vi "PlotBandsAgainstRun.vi"(8 "Bands?":bool, 11 "Graph":refnum<vi>) -> ()   [LabVIEW 2022 SP3]
panel:
  in  "Matlab":bool
  in  "Files":i32(listbox)
  in  "Stop Button":bool
  out "Data 2":cluster{dbl, "dt":dbl, "Y":dbl[]}[](graph)
  out "lines":i32
  out "Data":cluster{dbl, dbl, dbl[]}[](graph)
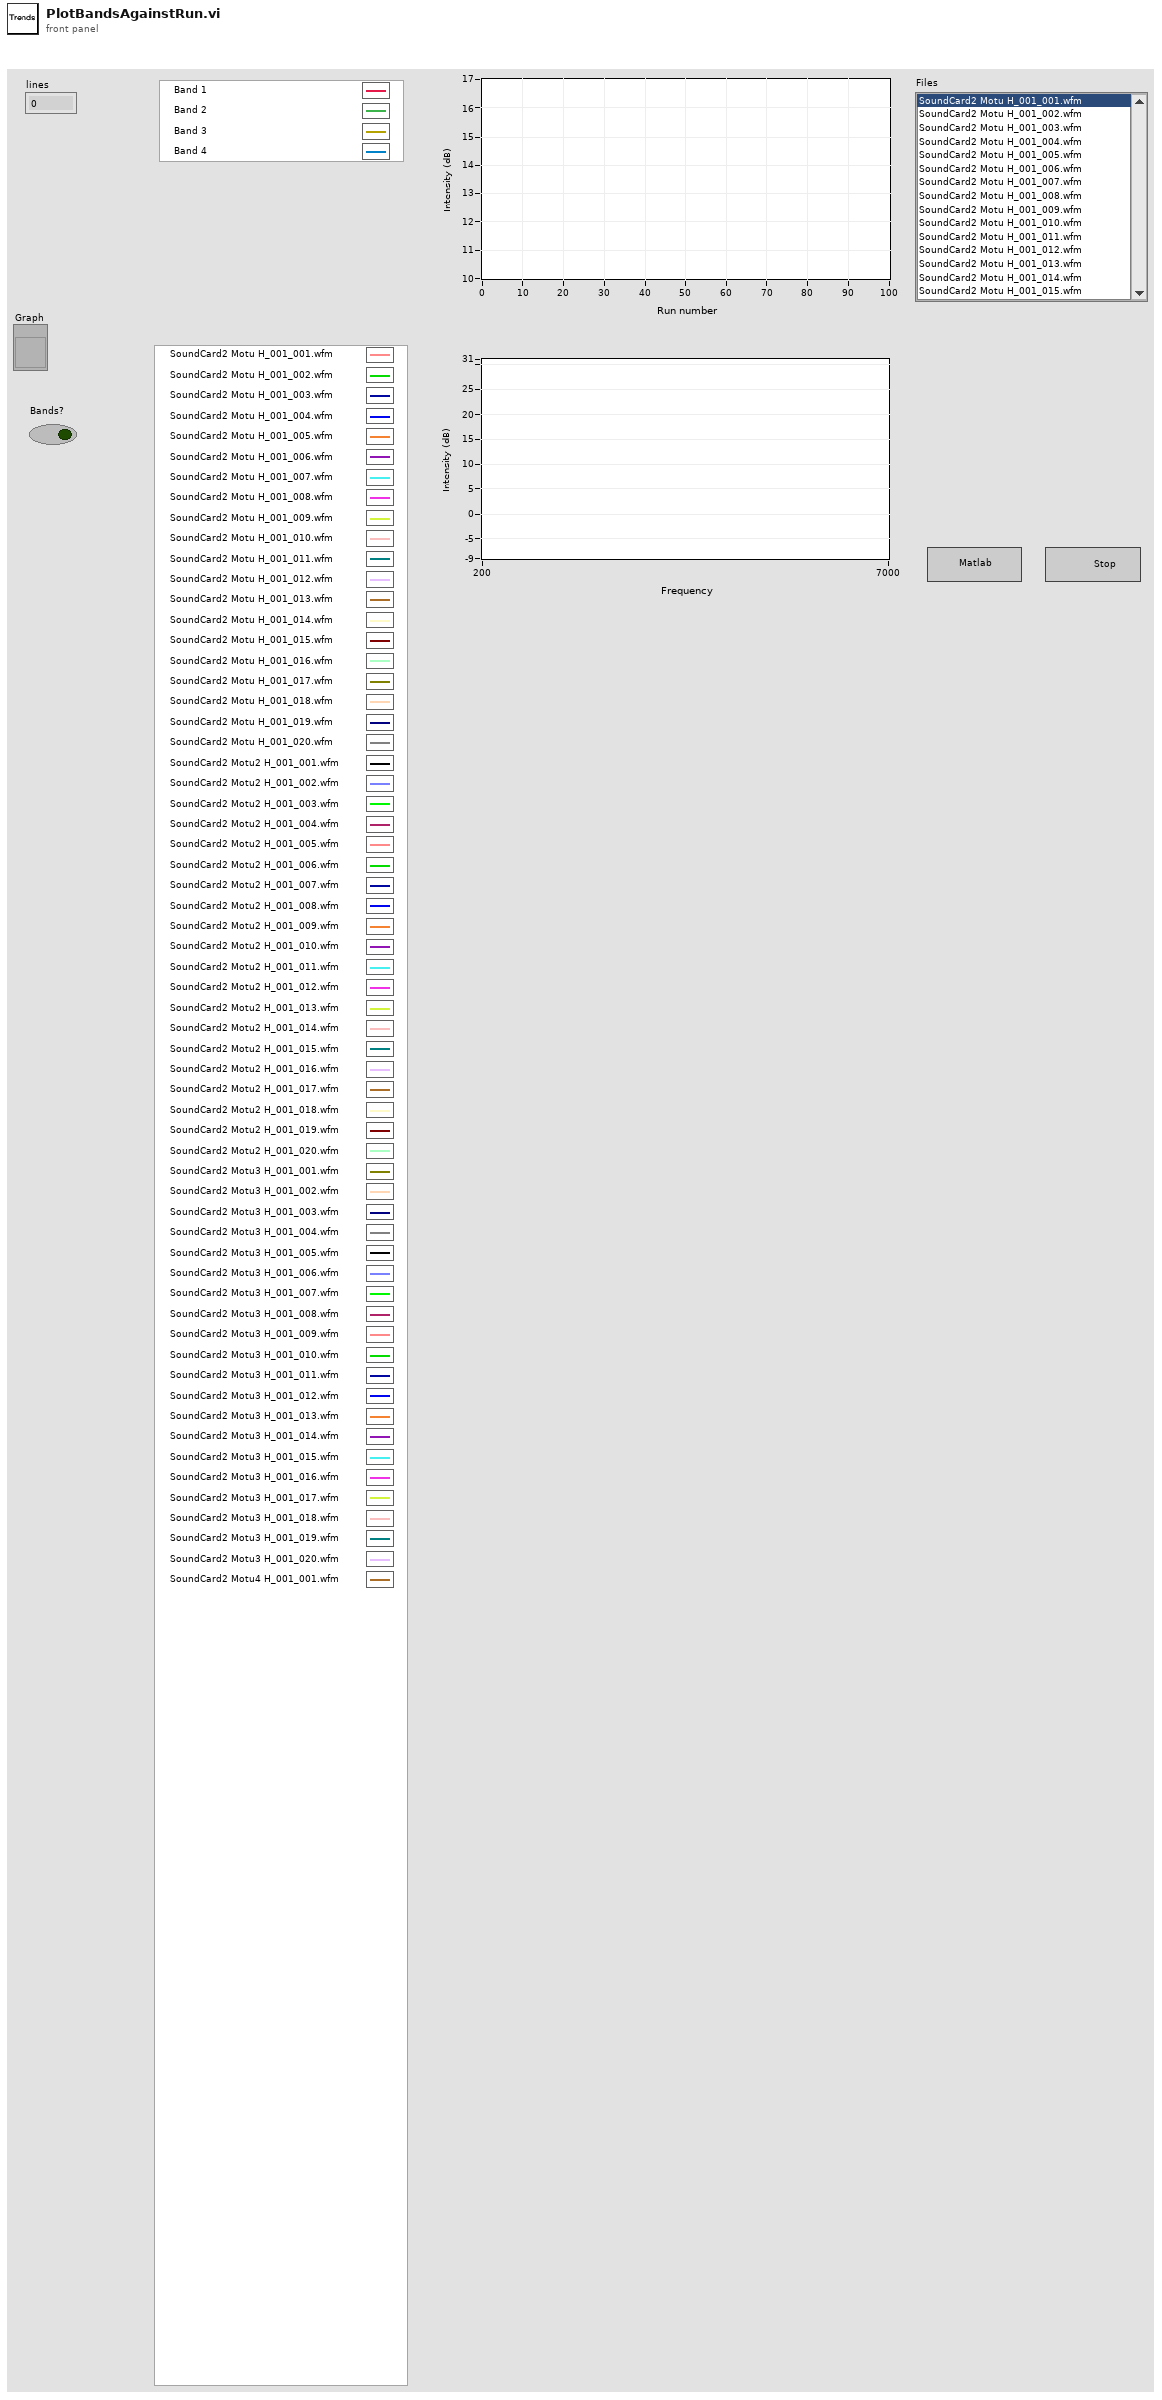
[diagram p1: front panel]
types:
  T1 = typedef "LVRangeTypeDef.ctl" = cluster{"Minimum":dbl, "Maximum":dbl, "Increment":dbl, "Minor Increment":dbl, "Start":dbl}
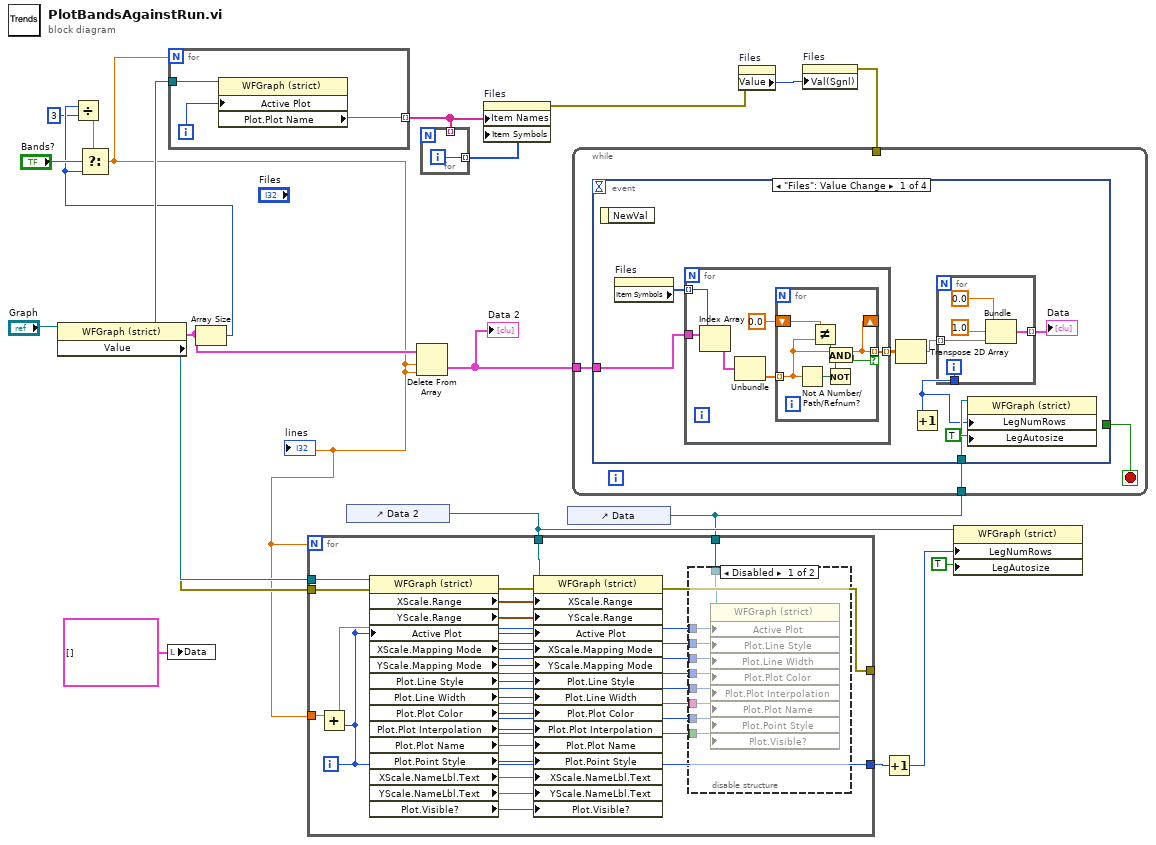
[diagram p0: block diagram]
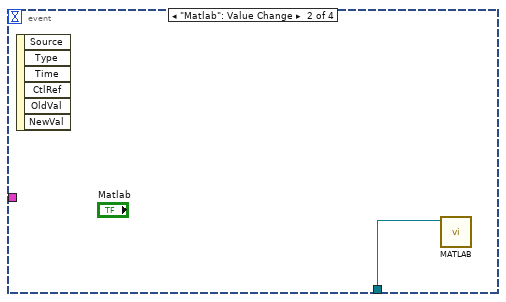
[diagram p3: hidden frame]
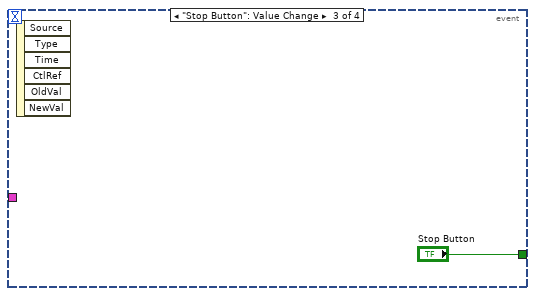
[diagram p4: hidden frame]
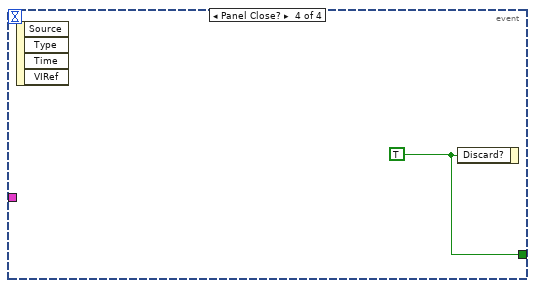
[diagram p5: hidden frame]
diagram:
  n1 = property class="WFGraph (strict)"(reference="Graph") -> (reference out=w11:refnum<vi>, error out=w10:errorcluster, "Value"=w20:cluster{dbl, "dt":dbl, "Y":dbl[]}[])  [unwired: 1 in]
  n2 = local write "Data"(cluster{dbl, dbl, dbl[]}[] [] ("Data")) -> ()
  n3 = Array Size(array=w20) -> (size(s)=w18:i32)
  n4 = Divide(x=w18, y=3) -> (x/y=w17:dbl)
  n5 = Select(t=w17, s="Bands?", f=w18) -> (s? t:f=w6:dbl)
  "lines" <- w6
  n6 = for {
    N: w6 -> [_]
    tunnel: "Graph" -> [w24]
    tunnel: [w22] -> w15 mode=indexing
    i -> [w23]
    n7 = property class="WFGraph (strict)"(reference=w24, "Active Plot"=w23) -> ("Plot.Plot Name"=w22:string)  [unwired: 1 in, 2 out]
  }
  n8 = control-ref of="Data 2"() -> (w4:refnum<vi>)
  n9 = Delete From Array(array=w20, length=w6, index=w6) -> (deleted portion=w9:cluster{dbl, "dt":dbl, "Y":dbl[]}[])  [unwired: 1 out]
  "Data 2" <- w9
  n10 = for {
    tunnel: w15 -> [_] mode=indexing
    tunnel: [w25] -> w14 mode=indexing
    i -> [w25]
  }
  n11 = property on="Files" class="LstBox (strict)"("Item Names"=w15, "Item Symbols"=w14) -> (error out=w12:errorcluster)  [unwired: 2 in, 1 out]
  n12 = control-ref of="Data"() -> (w2:refnum<vi>)
  n13 = for {
    N: w6 -> [_]
    tunnel: w11 -> [w46]
    tunnel: w10 -> [w45]
    tunnel: [w44] -> _
    tunnel: w6 -> [w43]
    tunnel: w4 -> [w28]
    tunnel: w2 -> [w27]
    tunnel: [w26] -> w7
    i -> [w26]
    n14 = Add(x=w43, y=w26) -> (x+y=w42:dbl)
    n15 = property class="WFGraph (strict)"(reference=w46, error in=w45, "Active Plot"=w42) -> (error out=w47:errorcluster, "XScale.Range"=w41:T1, "YScale.Range"=w40:T1, "XScale.Mapping Mode"=w39:u8, "YScale.Mapping Mode"=w38:u8, "Plot.Line Style"=w37:u8, "Plot.Line Width"=w36:u8, "Plot.Plot Color"=w35:u32, "Plot.Plot Interpolation"=w34:u8, "Plot.Plot Name"=w33:string, "Plot.Point Style"=w32:u8, "XScale.NameLbl.Text"=w31:string, "YScale.NameLbl.Text"=w30:string, "Plot.Visible?"=w29:bool)  [unwired: 1 out]
    n16 = property class="WFGraph (strict)"(reference=w28, error in=w47, "XScale.Range"=w41, "YScale.Range"=w40, "Active Plot"=w26, "XScale.Mapping Mode"=w39, "YScale.Mapping Mode"=w38, "Plot.Line Style"=w37, "Plot.Line Width"=w36, "Plot.Plot Color"=w35, "Plot.Plot Interpolation"=w34, "Plot.Plot Name"=w33, "Plot.Point Style"=w32, "XScale.NameLbl.Text"=w31, "YScale.NameLbl.Text"=w30, "Plot.Visible?"=w29) -> (error out=w44:errorcluster)  [unwired: 1 out]
    n17 = disable-structure shown="Disabled" {
      disable-tunnel: w37 -> [w56 _]
      disable-tunnel: w36 -> [w55 _]
      disable-tunnel: w35 -> [w54 _]
      disable-tunnel: w34 -> [w53 _]
      disable-tunnel: w33 -> [w52 _]
      disable-tunnel: w32 -> [w51 _]
      disable-tunnel: w29 -> [w50 _]
      disable-tunnel: w27 -> [w49 _]
      disable-tunnel: w26 -> [w48 _]
      frame Disabled {
        n18 = property class="WFGraph (strict)"(reference=w49, "Active Plot"=w48, "Plot.Line Style"=w56, "Plot.Line Width"=w55, "Plot.Plot Color"=w54, "Plot.Plot Interpolation"=w53, "Plot.Plot Name"=w52, "Plot.Point Style"=w51, "Plot.Visible?"=w50) -> ()  [unwired: 1 in, 2 out]
      }
      frame Enabled {
      }
    }
  }
  n19 = property on="Files" class="LstBox (strict)"(error in=w12) -> ("Value"=w13:i32)  [unwired: 1 in, 2 out]
  n20 = property on="Files" class="LstBox (strict)"("Val(Sgnl)"=w13) -> (error out=w8:errorcluster)  [unwired: 2 in, 1 out]
  n21 = while {
    tunnel: w9 -> [w59]
    tunnel: w8 -> [_]
    tunnel: w2 -> [w57]
    stop <- w58 stop-if-true
    n22 = event shown="[0] \"Files\": Value Change" {
      selector: _ -> [_ _ _ _]
      dyn-events: _ -> [_ _ _ _]
      timeout: _ -> [_ _ _ _]
      tunnel: w59 -> [w65 _ _ _]
      tunnel: [_ _ "Stop Button" w87] -> w58
      tunnel: w57 -> [w61 w85 _ _]
      event "Files": Value Change {
        n23 = event-data() -> ()  [unwired: 1 in, 1 out]
        n24 = property on="Files" class="LstBox (strict)"() -> ("Item Symbols"=w66:i32[])  [unwired: 2 in, 2 out]
        n25 = for {
          tunnel: w66 -> [w73] mode=indexing
          tunnel: w65 -> [w78]
          tunnel: [w75] -> w64 mode=indexing
          n26 = Index Array(array=w78, index=w73) -> (element=w77:cluster{dbl, "dt":dbl, "Y":dbl[]})
          n27 = Unbundle(w77) -> ("Y"=w76:dbl[])  [unwired: 2 out]
          n28 = for {
            tunnel: w76 -> [w82] mode=indexing
            tunnel: [w82] -> w75 mode=indexing if=w79
            shift-right: [w82] -> _
            shift-left: 0.0 -> [w83]
            n29 = Not A Number/Path/Refnum?(number/path/refnum=w82) -> (NaN/Path/Refnum?=w84:bool)
            n30 = Not Equal?(x=w83, y=w82) -> (x != y?=w81:bool)
            n31 = Not(x=w84) -> (.not. x?=w80:bool)
            n32 = And(x=w81, y=w80) -> (x .and. y?=w79:bool)
          }
        }
        n33 = Transpose 2D Array(2D array=w64) -> (transposed array=w63:dbl[][])
        n34 = for {
          tunnel: w63 -> [w72] mode=indexing
          tunnel: [w69] -> w67 mode=indexing
          tunnel: [w68] -> w60
          i -> [w68]
          n35 = Bundle(0.0, 1.0, w72) -> (w69:cluster{dbl, dbl, dbl[]})  [unwired: 1 in]
        }
        "Data" <- w67
        n36 = Increment(x=w60) -> ()  [unwired: 1 out]
        n37 = property class="WFGraph (strict)"(reference=w61, "LegNumRows"=w60, "LegAutosize"=TRUE ("Legend:Autosize")) -> ()  [unwired: 1 in, 2 out]
      }
      event "Matlab": Value Change {
        n38 = event-data() -> ()  [unwired: 1 in, 6 out]
        n39 = call "MATLAB.vi"("Graph"=w85) -> ()  [unwired: 10 in, 1 out]
      }
      event "Stop Button": Value Change {
        n40 = event-data() -> ()  [unwired: 1 in, 6 out]
      }
      event Panel Close? {
        w87 = TRUE ("Discard?")
        n41 = event-data() -> ()  [unwired: 1 in, 4 out]
        n42 = event-data("Discard?"=w87) -> ()  [unwired: 1 in, 1 out]
      }
    }
  }
  n43 = Increment(x=w7) -> (x+1=w3:i32)
  n44 = property class="WFGraph (strict)"(reference=w4, "LegNumRows"=w3, "LegAutosize"=TRUE ("Legend:Autosize")) -> ()  [unwired: 1 in, 2 out]
